vi "ServerTest.vi"() -> ()   [LabVIEW 2014]
panel:
  out "data out 2":string
  out "data out":string
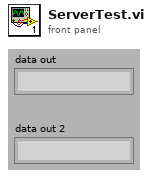
[diagram p1: front panel]
types:
  T1 = enum16{"Standard", "Buffered", "CRLF", "Immediate"}
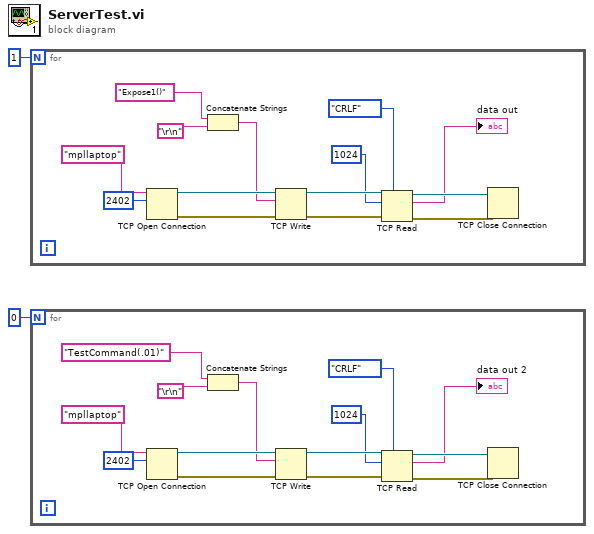
[diagram p0: block diagram]
diagram:
  n1 = for {
    N: 1 -> [_]
    n2 = TCP Open Connection(address="mpllaptop", remote port or service name=u16 2402) -> (connection ID=w16:refnum<k5>, error out=w13:errorcluster)  [unwired: 3 in]
    n3 = Concatenate Strings("Expose1()" ("data in"), "\r\n") -> (w3:string)
    n4 = TCP Write(connection ID=w16, data in=w3, error in (no error)=w13) -> (connection ID out=w14:refnum<k5>, error out=w12:errorcluster)  [unwired: 1 in, 1 out]
    n5 = TCP Read(connection ID=w14, bytes to read=1024, error in (no error)=w12, 7:T1."CRLF" ("mode (standard)")) -> (connection ID out=w15:refnum<k5>, data out=→"data out":string, error out=w11:errorcluster)  [unwired: 1 in]
    n6 = TCP Close Connection(connection ID=w15, error in (no error)=w11) -> ()  [unwired: 1 in, 2 out]
  }
  n7 = for {
    N: 0 -> [_]
    n8 = TCP Open Connection(address="mpllaptop", remote port or service name=u16 2402) -> (connection ID=w30:refnum<k5>, error out=w27:errorcluster)  [unwired: 3 in]
    n9 = Concatenate Strings("TestCommand(.01)" ("data in"), "\r\n") -> (w17:string)
    n10 = TCP Write(connection ID=w30, data in=w17, error in (no error)=w27) -> (connection ID out=w28:refnum<k5>, error out=w26:errorcluster)  [unwired: 1 in, 1 out]
    n11 = TCP Read(connection ID=w28, bytes to read=1024, error in (no error)=w26, 7:T1."CRLF" ("mode (standard)")) -> (connection ID out=w29:refnum<k5>, data out=→"data out 2":string, error out=w25:errorcluster)  [unwired: 1 in]
    n12 = TCP Close Connection(connection ID=w29, error in (no error)=w25) -> ()  [unwired: 1 in, 2 out]
  }
